vi "COMMUNICATION_SETTING.vi"(8 "error in":errorcluster, 11 "STATION":string) -> (0 "error out":errorcluster, 3 "COM":string)   [LabVIEW 2017]
uses:
  <vilib>/Utility/config.llb/Read Key (String).vi
  <vilib>/Utility/config.llb/NI_LVConfig.lvlib
panel:
  # "COMMUNICATION SETTING"
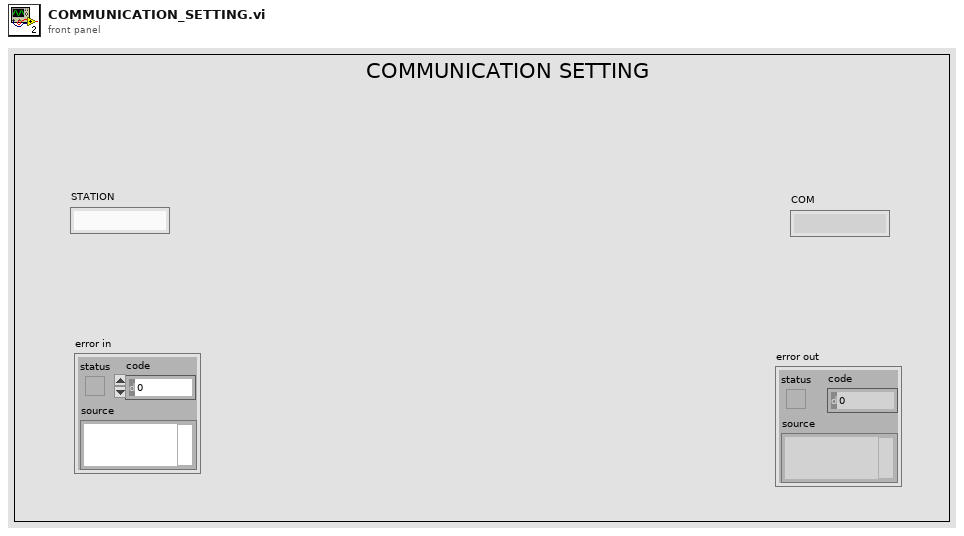
[diagram p1: front panel]
types:
  T1 = enum32{"invalid app kind", "Development System", "Run Time System", "Student Edition", "Embedded LabVIEW", "Evaluation", "Custom"}
  T2 = typedef "NI_LVConfig.lvlib/Config Data RefNum.ctl" = refnum<k1>
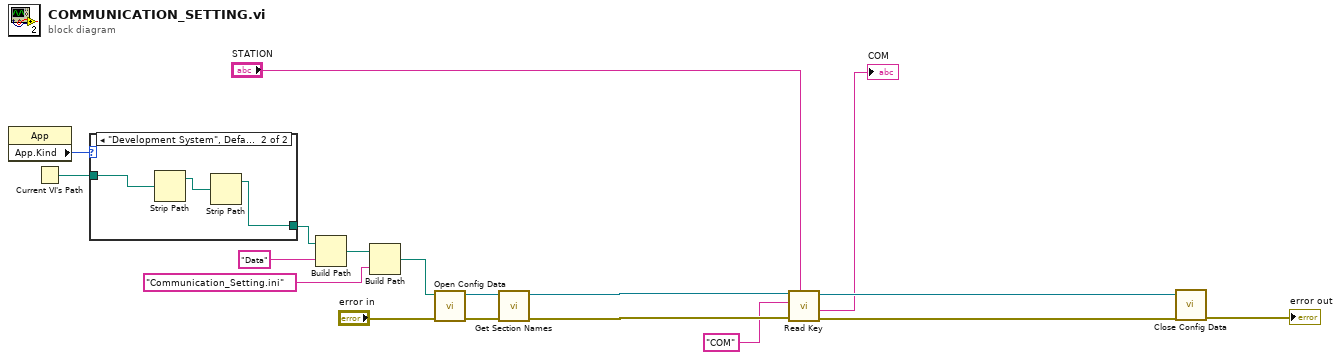
[diagram p0: block diagram]
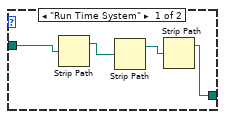
[diagram p2: hidden frame]
diagram:
  n1 = property class="App"() -> ("App.Kind"=w17:T1)  [unwired: 2 in, 2 out]
  n2 = Current VI's Path() -> (path=w18:path)
  n3 = case shown="\"Development System\", Default" w17 {
    tunnel: w18 -> [w20 w24]
    tunnel: [w19 w23] -> w15
    frame "Run Time System" {
      n4 = Strip Path(path=w20) -> (stripped path=w22:path)  [unwired: 1 out]
      n5 = Strip Path(path=w22) -> (stripped path=w21:path)  [unwired: 1 out]
      n6 = Strip Path(path=w21) -> (stripped path=w19:path)  [unwired: 1 out]
    }
    frame "Development System", Default {
      n7 = Strip Path(path=w24) -> (stripped path=w25:path)  [unwired: 1 out]
      n8 = Strip Path(path=w25) -> (stripped path=w23:path)  [unwired: 1 out]
    }
  }
  n9 = Build Path(base path=w15, name or relative path="Data") -> (appended path=w16:path)
  n10 = Build Path(base path=w16, name or relative path="Communication_Setting.ini") -> (appended path=w14:path)
  n11 = call <vilib>:"Open Config Data.vi"("error in (no error)"="error in", "configuration file path"=w14) -> ("error out"=w10:errorcluster, "refnum"=w11:T2)  [unwired: 7 in, 1 out]
  n12 = call <vilib>:"Get Section Names.vi"("error in (no error)"=w10, "refnum"=w11) -> ("error out"=w7:errorcluster, "refnum out"=w6:T2)  [unwired: 7 in, 1 out]
  n13 = call-poly <vilib>:"Read Key.vi"("section"="STATION", "error in (no error)"=w7, "key"="COM" ("name or relative path"), "refnum"=w6) -> ("error out"=w5:errorcluster, "value"=→"COM":string, "refnum out"=w4:T2)  [unwired: 4 in, 1 out]
  n14 = call <vilib>:"Close Config Data.vi"("error in (no error)"=w5, "refnum"=w4) -> ("error out"=→"error out":errorcluster)  [unwired: 8 in, 1 out]
